vi "VI Front Panel Items Map.vi"(8 "error in (no error)":errorcluster, 11 "VI in":refnum<vi>) -> (0 "error out":errorcluster, 3 "Map":map{string, refnum<vi>}(c390))   [LabVIEW 2026, in "TALOS.lvlib" / "Father of all uServices.lvlib" / "Father of all uServices.lvclass"]
uses:
  Father of all uServices.lvclass
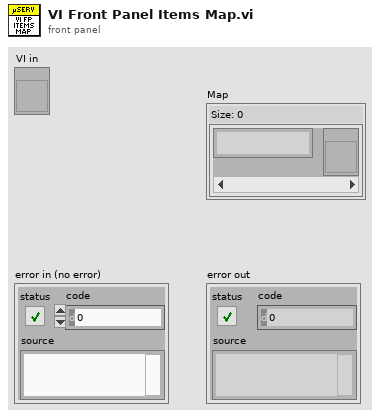
[diagram p1: front panel]
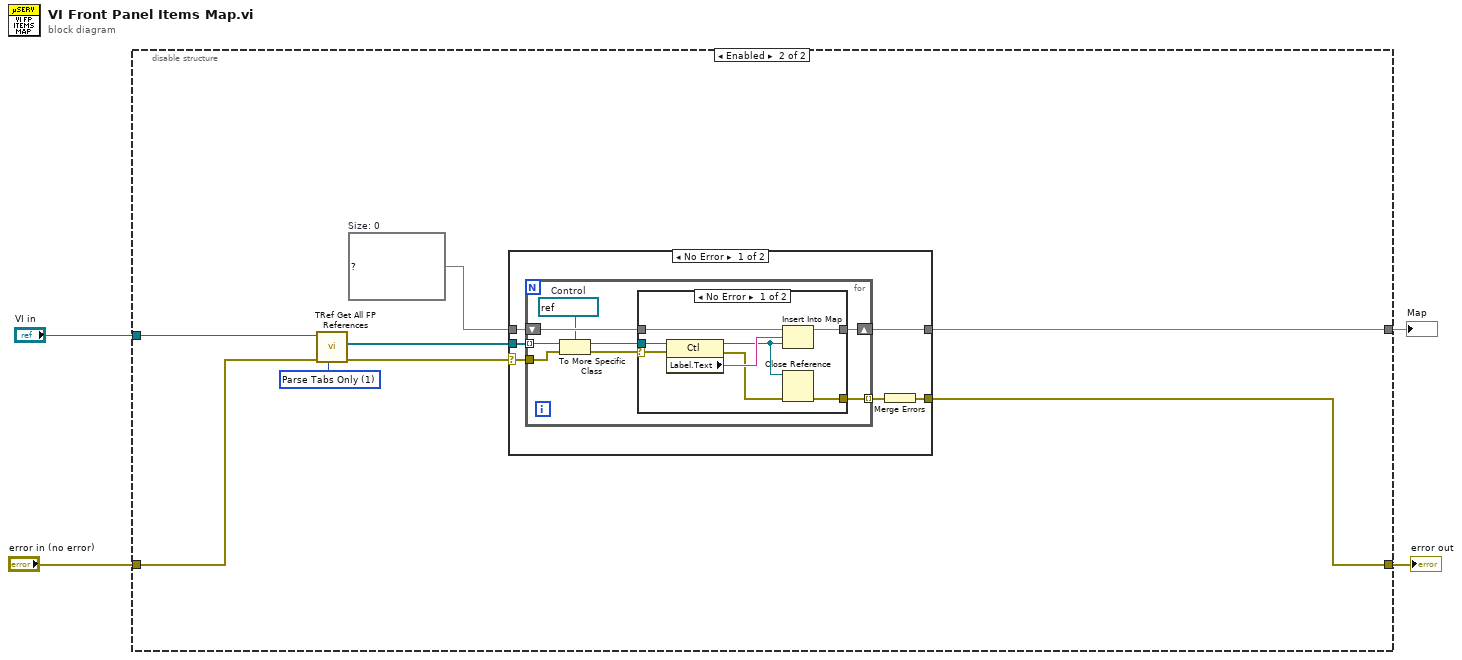
[diagram p0: block diagram]
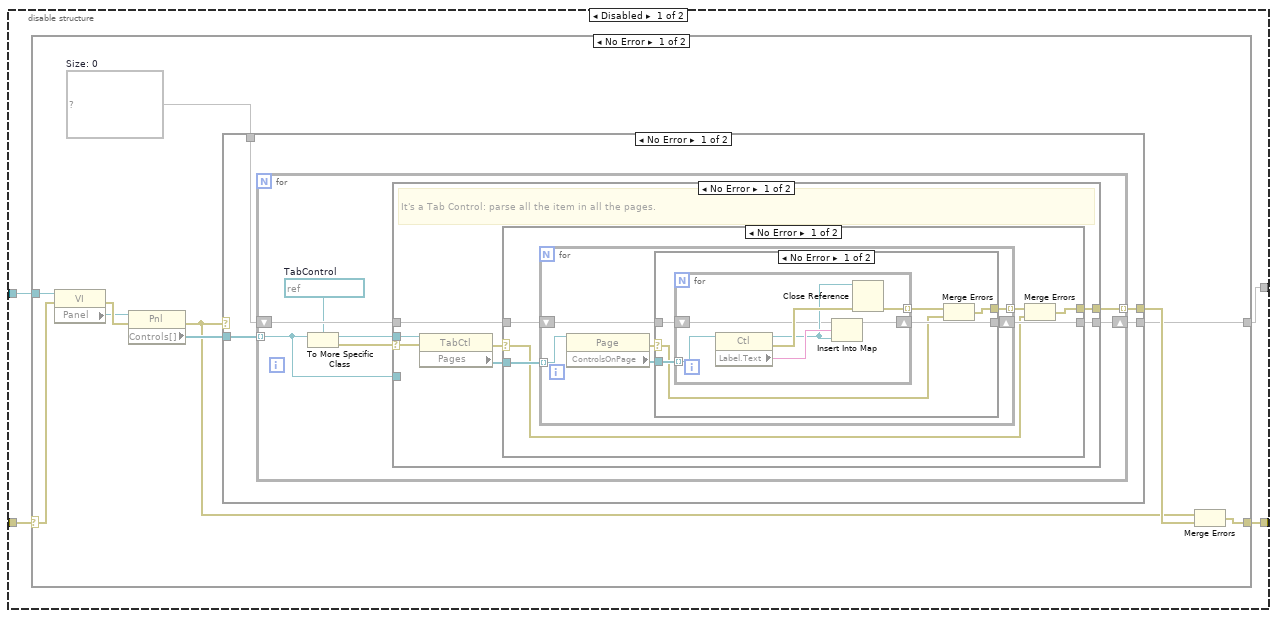
[diagram p2: hidden frame]
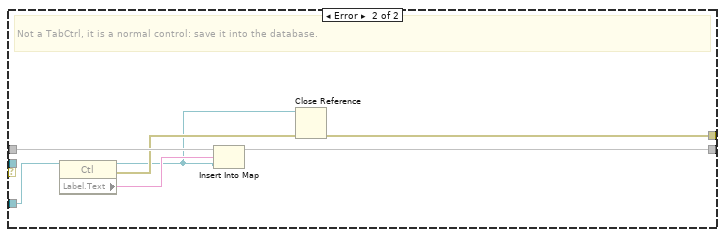
[diagram p5: hidden frame]
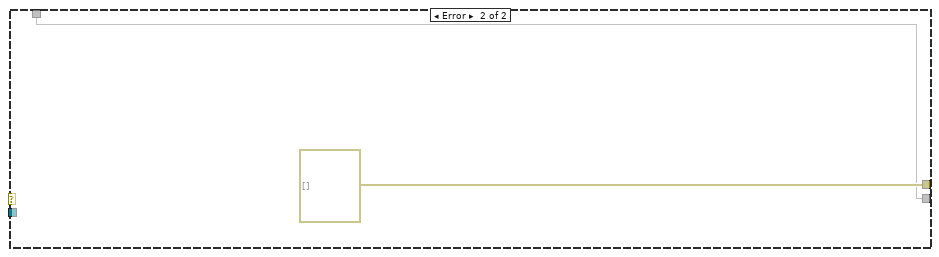
[diagram p6: hidden frame]
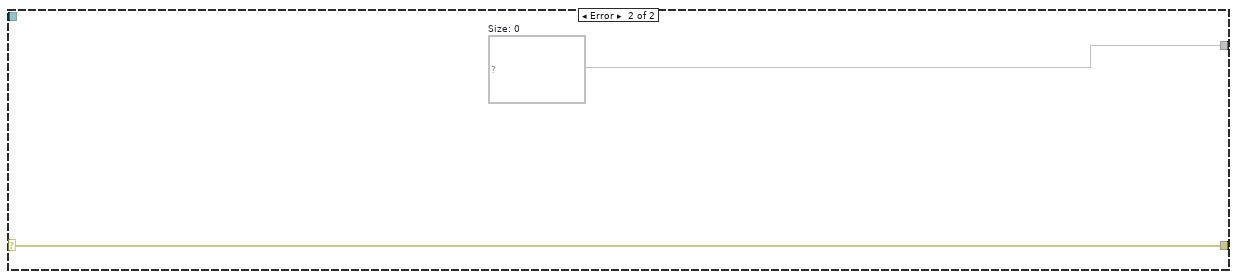
[diagram p7: hidden frame]
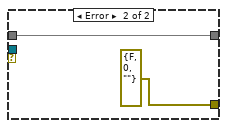
[diagram p8: hidden frame]
diagram:
  n1 = disable-structure shown="Enabled" {
    disable-tunnel: "VI in" -> [w8 w83]
    disable-tunnel: [w7 w78] -> w3
    disable-tunnel: "error in (no error)" -> [w6 w82]
    disable-tunnel: [w5 w79] -> w1
    frame Disabled {
      n2 = case shown="No Error" w6 {
        selector: w6 -> [w11 w76]
        tunnel: w8 -> [w18 _]
        tunnel: [w16 w76] -> w7
        tunnel: [w10 w75] -> w5
        frame No Error {
          w17 = map{string, refnum<vi>} {}  # Size: 0
          n3 = property on="Property Node" class="VI"(reference=w18, error in=w11) -> (error out=w14:errorcluster, "Panel"=w12:refnum<vi>)  [unwired: 1 out]
          n4 = property on="Property Node" class="Pnl"(reference=w12, error in=w14) -> (error out=w9:errorcluster, "Controls[]"=w13:refnum<vi>[])  [unwired: 1 out]
          n5 = case shown="No Error" w9 {
            tunnel: w17 -> [w22 w73]
            tunnel: [w21 errorcluster[] []] -> w15
            tunnel: w13 -> [w20 _]
            tunnel: [w19 w73] -> w10
            frame No Error {
              n6 = for {
                tunnel: w20 -> [w23] mode=indexing
                shift-right: [w29] -> w19
                shift-left: w22 -> [w28]
                tunnel: [w27] -> w21 mode=indexing
                w25 = refnum<vi> refnum  # TabControl
                n7 = To More Specific Class(target class=w25, reference=w23) -> (specific class reference=w26:refnum<vi>, error out=w24:errorcluster)  [unwired: 1 in]
                n8 = case shown="No Error" w24 {
                  selector: w24 -> [w35 _]
                  tunnel: [w31 w71] -> w29
                  tunnel: w28 -> [w32 w70]
                  tunnel: [w30 w68] -> w27
                  tunnel: w26 -> [w36 _]
                  tunnel: w23 -> [_ w66]
                  frame No Error {
                    # "It's a Tab Control: parse all the item in all the pages."
                    n9 = property on="Property Node" class="TabCtl"(reference=w36, error in=w35) -> (error out=w33:errorcluster, "Pages"=w34:refnum<vi>[])  [unwired: 1 out]
                    n10 = case shown="No Error" w33 {
                      selector: w33 -> [w37 w64]
                      tunnel: w34 -> [w42 _]
                      tunnel: w32 -> [w41 w65]
                      tunnel: [w40 w65] -> w31
                      tunnel: [w39 w64] -> w30
                      frame No Error {
                        n11 = for {
                          tunnel: w42 -> [w48] mode=indexing
                          shift-right: [w45] -> w40
                          shift-left: w41 -> [w46]
                          tunnel: [w43] -> w38 mode=indexing
                          n12 = property on="Property Node" class="Page"(reference=w48) -> (error out=w44:errorcluster, "ControlsOnPage"=w47:refnum<vi>[])  [unwired: 1 in, 1 out]
                          n13 = case shown="No Error" w44 {
                            selector: w44 -> [w49 w63]
                            tunnel: w47 -> [w54 _]
                            tunnel: w46 -> [w53 w62]
                            tunnel: [w52 w62] -> w45
                            tunnel: [w50 w63] -> w43
                            frame No Error {
                              n14 = for {
                                tunnel: w54 -> [w56] mode=indexing
                                shift-right: [w57] -> w52
                                shift-left: w53 -> [w58]
                                tunnel: [w55] -> w51 mode=indexing
                                n15 = property on="Property Node" class="Ctl"(reference=w56) -> (reference out=w59:refnum<vi>, error out=w60:errorcluster, "Label.Text"=w61:string)  [unwired: 1 in]
                                n16 = Insert Into Map(map in=w58, key=w61, value=w59) -> (map out=w57:map{string, refnum<vi>})  [unwired: 2 out]
                                n17 = Close Reference(reference=w59, error in (no error)=w60) -> (error out=w55:errorcluster)
                              }
                              n18 = Merge Errors(w51, w49) -> (w50:errorcluster)
                            }
                            frame Error {
                            }
                          }
                        }
                        n19 = Merge Errors(w38, w37) -> (w39:errorcluster)
                      }
                      frame Error {
                      }
                    }
                  }
                  frame Error {
                    # "Not a TabCtrl, it is a normal control: save it into the database."
                    n20 = property on="Property Node" class="Ctl"(reference=w66) -> (reference out=w67:refnum<vi>, error out=w69:errorcluster, "Label.Text"=w72:string)  [unwired: 1 in]
                    n21 = Insert Into Map(map in=w70, key=w72, value=w67) -> (map out=w71:map{string, refnum<vi>})  [unwired: 2 out]
                    n22 = Close Reference(reference=w67, error in (no error)=w69) -> (error out=w68:errorcluster)
                  }
                }
              }
            }
            frame Error {
            }
          }
          n23 = Merge Errors(w9, w15) -> (w16:errorcluster)
        }
        frame Error {
          w75 = map{string, refnum<vi>} {}  # Size: 0
        }
      }
    }
    frame Enabled {
      w81 = map{string, refnum<vi>} {}  # Size: 0
      w84 = u16 1 items=["Parse All", "Parse Tabs Only"] ("Parsing Rule")
      n24 = call <vilib>:"TRef Get All FP References.vi"("Parsing Rule"=w84, "error in (no error)"=w82, "VI Refnum"=w83) -> ("error out"=w77:errorcluster, "All FP Objects"=w80:refnum<vi>[])  [unwired: 4 in, 3 out]
      n25 = case shown="No Error" w77 {
        selector: w77 -> [w85 w109]
        tunnel: w81 -> [w90 w110]
        tunnel: w80 -> [w89 _]
        tunnel: [w88 w110] -> w79
        tunnel: [w86 w109] -> w78
        frame No Error {
          n26 = for {
            tunnel: w89 -> [w94] mode=indexing
            shift-right: [w97] -> w88
            shift-left: w90 -> [w98]
            tunnel: [w96] -> w87 mode=indexing
            tunnel: w85 -> [w93]
            w95 = refnum<vi> refnum  # Control
            n27 = To More Specific Class(target class=w95, reference=w94, error in=w93) -> (specific class reference=w92:refnum<vi>, error out=w91:errorcluster)
            n28 = case shown="No Error" w91 {
              selector: w91 -> [w99 _]
              tunnel: w98 -> [w103 w108]
              tunnel: [w102 w108] -> w97
              tunnel: [w101 errorcluster {"status"=FALSE, "code"=0, "source"=""} ("error out")] -> w96
              tunnel: w92 -> [w100 _]
              frame No Error {
                n29 = property on="Property Node" class="Ctl"(reference=w100, error in=w99) -> (reference out=w104:refnum<vi>, error out=w105:errorcluster, "Label.Text"=w106:string)
                n30 = Insert Into Map(map in=w103, key=w106, value=w104) -> (map out=w102:map{string, refnum<vi>})  [unwired: 2 out]
                n31 = Close Reference(reference=w104, error in (no error)=w105) -> (error out=w101:errorcluster)
              }
              frame Error {
              }
            }
          }
          n32 = Merge Errors(w87) -> (w86:errorcluster)
        }
        frame Error {
        }
      }
    }
  }
  "error out" <- w3
  "Map" <- w1
